vi "Read Field name.vi"(8 "error in (no error)":errorcluster, 11 "Write FP Control Msg in":refnum<class "Write FP Control Msg.lvclass">) -> (0 "error out":errorcluster, 2 "Field name":string, 3 "Write FP Control Msg out":refnum<class "Write FP Control Msg.lvclass">)   [LabVIEW 2016, in "Write FP Control Msg.lvclass"]
uses:
  Write FP Control Msg.lvclass
  Write FP Control Msg.lvclass/Write FP Control Msg.ctl
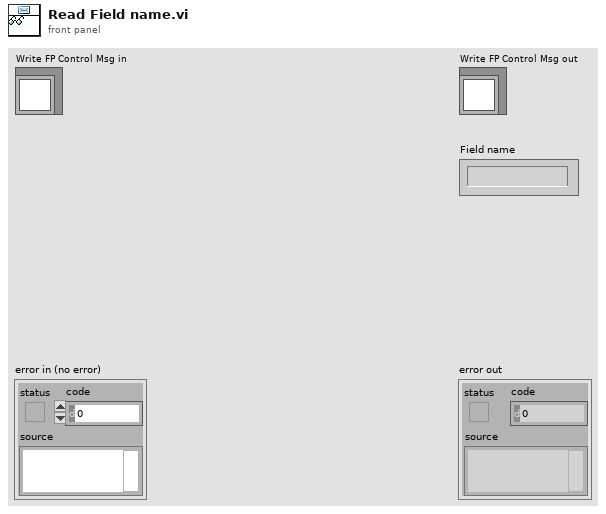
[diagram p1: front panel]
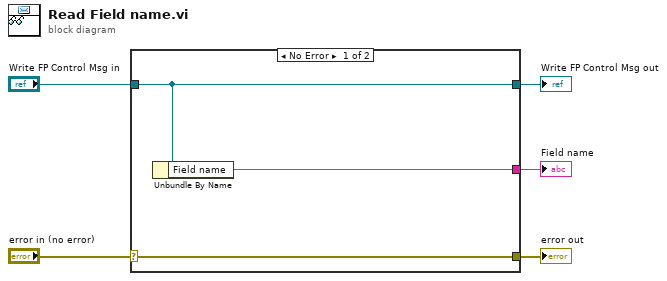
[diagram p0: block diagram]
diagram:
  n1 = case shown="No Error" "error in (no error)" {
    selector: "error in (no error)" -> [w8 w9]
    tunnel: [w8 w9] -> w4
    tunnel: [w7 w10] -> w2
    tunnel: "Write FP Control Msg in" -> [w7 w10]
    tunnel: [w6 _] -> w1
    frame No Error {
      n2 = Unbundle By Name(w7) -> ("Field name"=w6:string)
    }
    frame Error {
    }
  }
  "error out" <- w4
  "Write FP Control Msg out" <- w2
  "Field name" <- w1
